vi "Data_LoadPictureByPath.vi"(8 "error in (no error)":errorcluster caption="错误输入（无错误）", 10 "Image Path":path, 11 "Picture_Class 输入":refnum<class "Picture_Class.lvclass"> caption="DNL_LabVIEW Object in") -> (0 "error out":errorcluster caption="错误输出", 3 "Picture_Class 输出":refnum<class "Picture_Class.lvclass"> caption="DNL_LabVIEW Object out")   [LabVIEW 2013, in "Picture_Class.lvclass"]
uses:
  Picture_Class.lvclass
  Picture_Class.lvclass/Picture_Class.ctl
  <vilib>/Utility/error.llb/DialogType.ctl
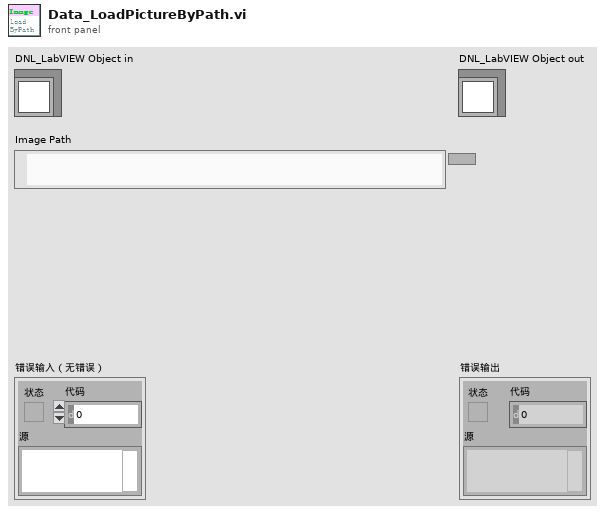
[diagram p1: front panel]
types:
  T1 = typedef "DialogType.ctl" = u16
  T2 = typedef "imagedata.ctl" = cluster{"image type":i32, "image depth":i32, "image":u8[], "mask":u8[], "colors":u32[], "Rectangle":cluster{"left":i16, "top":i16, "right":i16, "bottom":i16}}
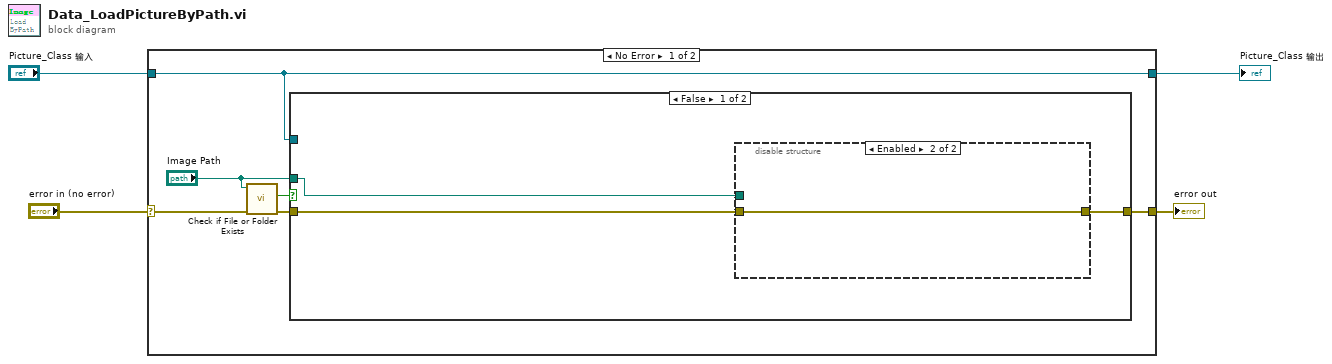
[diagram p0: block diagram]
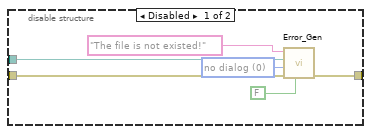
[diagram p2: hidden frame]
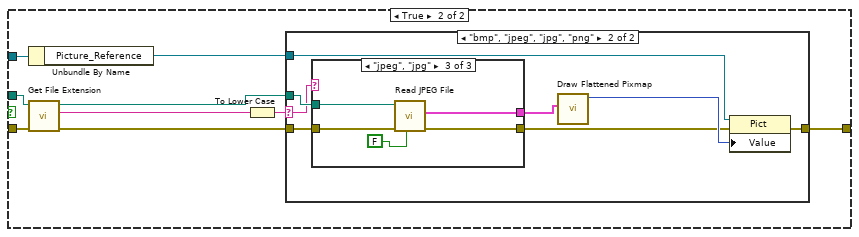
[diagram p3: hidden frame]
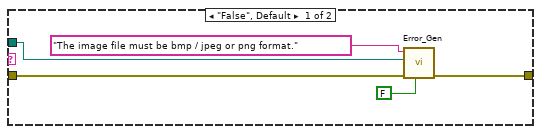
[diagram p4: hidden frame]
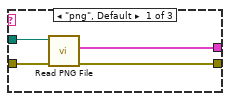
[diagram p5: hidden frame]
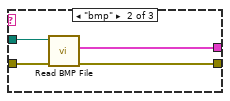
[diagram p6: hidden frame]
diagram:
  n1 = case shown="No Error" "error in (no error)" {
    selector: "error in (no error)" -> [w7 w57]
    tunnel: [w9 w57] -> w3
    tunnel: [w10 w56] -> w1
    tunnel: "Picture_Class 输入" -> [w10 w56]
    frame No Error {
      n2 = call <vilib>:"Check if File or Folder Exists.vi"("error in (no error)"=w7, "path"="Image Path") -> ("error out"=w5:errorcluster, "file or folder exists?"=w6:bool)  [unwired: 7 in, 1 out]
      n3 = case shown="False" w6 {
        tunnel: w10 -> [_ w29]
        tunnel: [w12 w28] -> w9
        tunnel: "Image Path" -> [w11 w23]
        tunnel: w5 -> [w13 w25]
        frame False {
          n4 = disable-structure shown="Enabled" {
            disable-tunnel: w13 -> [w19 w20]
            disable-tunnel: [w18 w20] -> w12
            disable-tunnel: w11 -> [w16 _]
            frame Disabled {
              w14 = T1 0 items=["no dialog", "OK message", "continue or stop message", "OK message + warnings", "continue/stop + warnings"] ("type of dialog (OK msg:1)")
              n5 = call "Error_Gen.vi"("Error(T)/Warning"=FALSE, "error in"=w19, "type of dialog (OK msg:1)"=w14, "ErrorInfor"=w16, "message"="The file is not existed!") -> ("error out"=w18:errorcluster)  [unwired: 6 in]
            }
            frame Enabled {
            }
          }
        }
        frame True {
          n6 = Unbundle By Name(w29) -> ("Picture_Reference"=w27:refnum<vi>)
          n7 = call <vilib>:"Get File Extension.vi"("error in (no error)"=w25, "file"=w23) -> ("error out"=w24:errorcluster, "lowercase file extension"=w26:string, "dup file"=w22:path)  [unwired: 6 in, 1 out]
          n8 = To Lower Case(string=w26) -> (all lower case string=w21:string)
          n9 = case shown="\"bmp\", \"jpeg\", \"jpg\", \"png\"" w21 {
            selector: w21 -> [_ w35]
            tunnel: [w31 w42] -> w28
            tunnel: w27 -> [_ w41]
            tunnel: w22 -> [w30 w37]
            tunnel: w24 -> [w32 w36]
            frame "False", Default {
              n10 = call "Error_Gen.vi"("Error(T)/Warning"=FALSE, "error in"=w32, "ErrorInfor"=w30, "message"="The image file must be bmp / jpeg or png format.") -> ("error out"=w31:errorcluster)  [unwired: 7 in]
            }
            frame "bmp", "jpeg", "jpg", "png" {
              n11 = case shown="\"jpeg\", \"jpg\"" w35 {
                tunnel: [w43 w47 w54] -> w40
                tunnel: [w45 w49 w53] -> w38
                tunnel: w37 -> [w44 w48 w52]
                tunnel: w36 -> [w46 w50 w51]
                frame "png", Default {
                  n12 = call <vilib>:"Read PNG File.vi"("error in (no error)"=w46, "path to PNG file"=w44) -> ("error out"=w45:errorcluster, "image data"=w43:T2)  [unwired: 7 in, 1 out]
                }
                frame "bmp" {
                  n13 = call <vilib>:"Read BMP File.vi"("error in (no error)"=w50, "path to BMP file"=w48) -> ("error out"=w49:errorcluster, "image data"=w47:T2)  [unwired: 7 in, 1 out]
                }
                frame "jpeg", "jpg" {
                  n14 = call <vilib>:"Read JPEG File.vi"("use 8 bit color table"=FALSE, "error in (no error)"=w51, "path to JPEG file"=w52) -> ("error out"=w53:errorcluster, "image data"=w54:T2)  [unwired: 6 in, 1 out]
                }
              }
              n15 = call <vilib>:"Draw Flattened Pixmap.vi"("image data"=w40) -> ("new picture"=w39:picture)  [unwired: 8 in]
              n16 = property class="Pict"(reference=w41, error in=w38, "Value"=w39) -> (error out=w42:errorcluster)  [unwired: 1 out]
            }
          }
        }
      }
    }
    frame Error {
    }
  }
  "error out" <- w3
  "Picture_Class 输出" <- w1
